vi "Read Exe Complete.vi"(8 "error in (no error)":errorcluster, 11 "GUI in":refnum<class "GUI.lvclass">) -> (0 "error out":errorcluster, 2 "Exe Complete?":refnum<notifier>, 3 "GUI out":refnum<class "GUI.lvclass">)   [LabVIEW 2018, in "GUI.lvclass"]
uses:
  GUI.lvclass
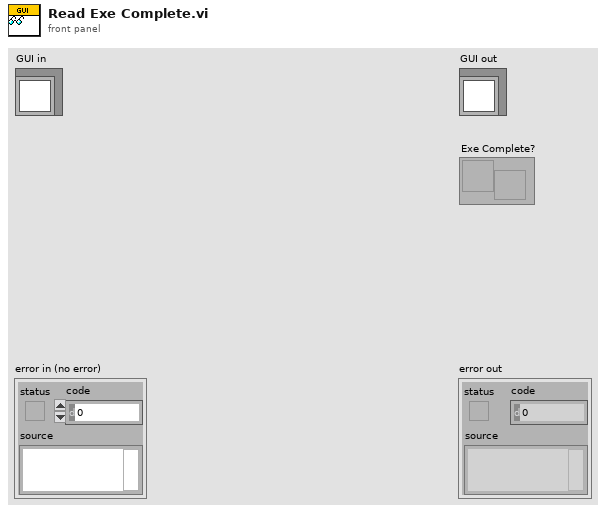
[diagram p1: front panel]
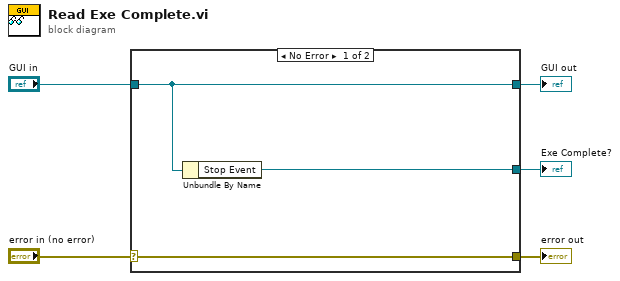
[diagram p0: block diagram]
diagram:
  n1 = case shown="No Error" "error in (no error)" {
    selector: "error in (no error)" -> [w8 w9]
    tunnel: [w8 w9] -> w4
    tunnel: [w7 w10] -> w2
    tunnel: "GUI in" -> [w7 w10]
    tunnel: [w6 _] -> w1
    frame No Error {
      n2 = Unbundle By Name(w7) -> ("Stop Event"=w6:refnum<user-event>)
    }
    frame Error {
    }
  }
  "error out" <- w4
  "GUI out" <- w2
  "Exe Complete?" <- w1
